vi "Get AsyncCommandQ Ref.vi"(11 "TimerDRV in":refnum<class "TimerDRV.lvclass">) -> (2 "AsyncCommandQ":refnum<queue>, 3 "TimerDRV out":refnum<class "TimerDRV.lvclass">)   [LabVIEW 2019, in "TimingDRV Engine.lvlib" / "TimerDRV.lvclass"]
uses:
  TimerDRV.lvclass
  TypeDefs/Command Package.ctl
  TypeDefs/Command.ctl
  TimerDRV.lvclass/TimerDRV.ctl
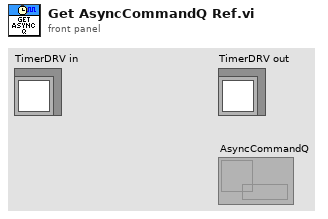
[diagram p1: front panel]
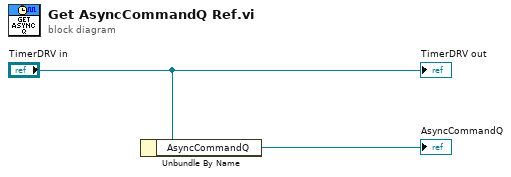
[diagram p0: block diagram]
diagram:
  n1 = Unbundle By Name("TimerDRV in") -> ("AsyncCommandQ"=→"AsyncCommandQ":refnum<queue>)
  "TimerDRV out" <- "TimerDRV in"
